vi "分层图显示1.2.1（导入色码表）.vi"(11 "IN":string) -> (3 "OUT":string)   [LabVIEW 2016]
uses:
  <vilib>/Utility/file.llb/Read Delimited Spreadsheet (DBL).vi
  <vilib>/Utility/file.llb/Read Delimited Spreadsheet (I64).vi
panel:
  in  "更换色码":bool
  in  "色码表导入":path=path "C:/Users/H301/Desktop/art闭环扫描程序/色码表/色码表（彩色2）.txt" caption="（色码表导入）"
  out "导入进度":u8(slide) scale=0.0..100.0
  in  "min":dbl format="%#_4e"
  in  "max":dbl format="%#_4e"
  in  "ESC":bool
  out "分层图":dbl[][](graph)
  in  "NEXT":bool
  in  "层数:":i32
  out "数组":dbl[][][](array[numeric])
  # "强度表"
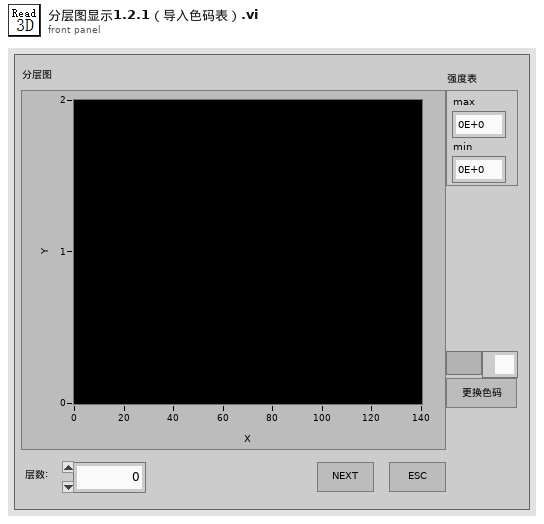
[diagram p1: front panel]
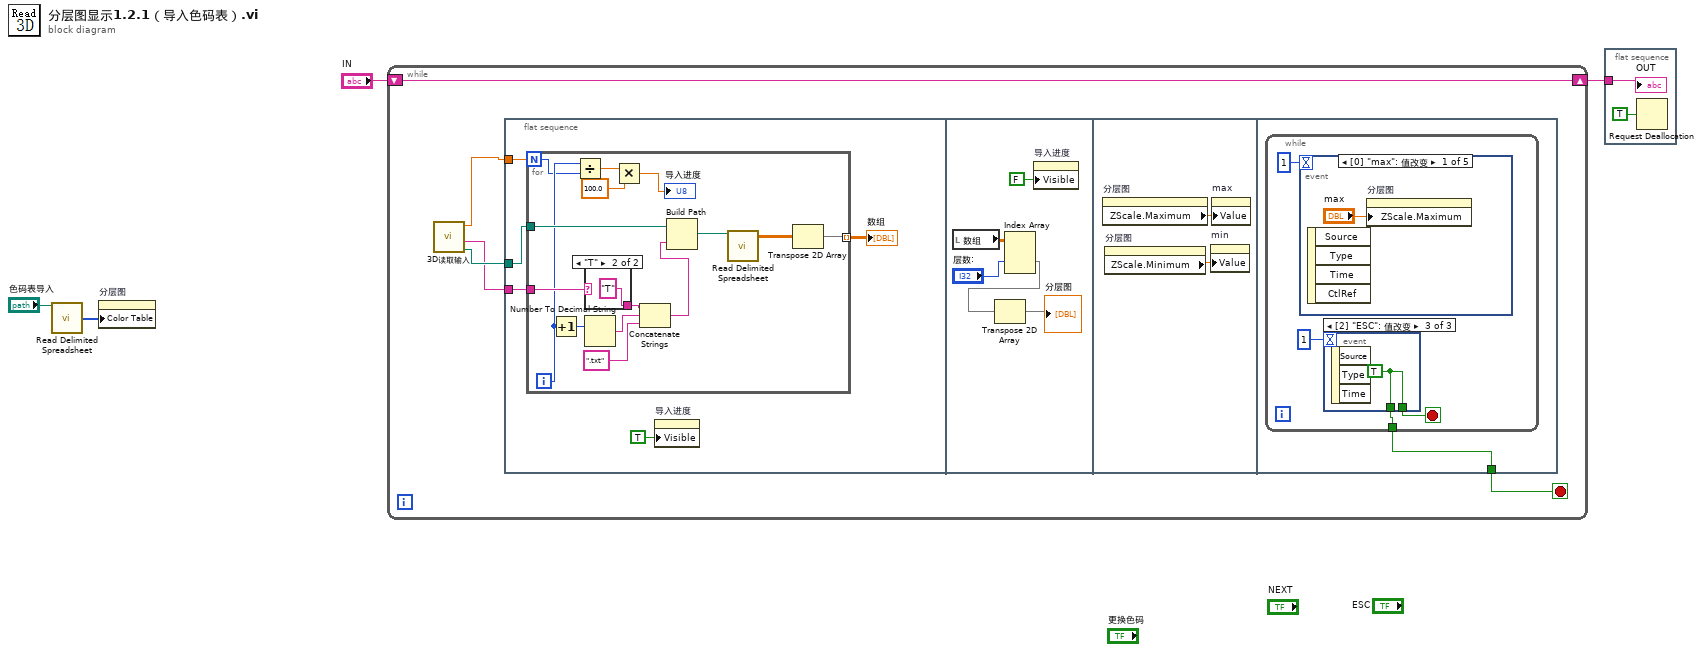
[diagram p0: block diagram]
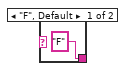
[diagram p2: hidden frame]
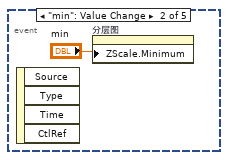
[diagram p3: hidden frame]
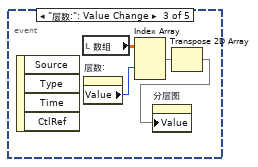
[diagram p4: hidden frame]
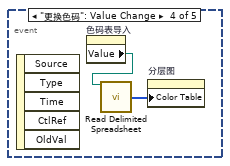
[diagram p5: hidden frame]
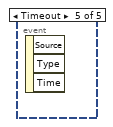
[diagram p6: hidden frame]
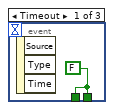
[diagram p7: hidden frame]
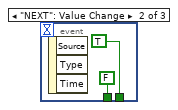
[diagram p8: hidden frame]
diagram:
  n1 = call-poly <vilib>:"Read Delimited Spreadsheet.vi"("file path (dialog if empty)"="色码表导入") -> ("first row"=w2:i64[])  [unwired: 9 in, 5 out]
  n2 = property on="分层图" class="IntGraph (严格)"("Color Table"=w2) -> ()  [unwired: 2 in, 2 out]
  n3 = while {
    shift-right: [w9] -> w3
    shift-left: "IN" -> [w9]
    stop <- w8 stop-if-true
    n4 = call "3D读取输入.vi"() -> ("文件读取路径"=w6:path, "时域谱or频域谱"=w5:string, "行总数"=w7:dbl)  [unwired: 9 in]
    n5 = flat-sequence {
      tunnel: w7 -> [w13]
      tunnel: w5 -> [w12]
      tunnel: w6 -> [w11]
      tunnel: [w39] -> w8
      frame #0 {
        n6 = for {
          N: w13 -> [w18]
          tunnel: [w28] -> w14 mode=indexing
          tunnel: w12 -> [w21]
          tunnel: w11 -> [w20]
          i -> [w19]
          n7 = Increment(x=w19) -> (x+1=w24:i32)
          n8 = Divide(x=w19, y=w18) -> (x/y=w17:dbl)
          n9 = case shown="\"T\"" w21 {
            tunnel: ["F" "T"] -> w26
            frame "F", Default {
            }
            frame "T" {
            }
          }
          n10 = Number To Decimal String(number=w24) -> (decimal integer string=w23:string)  [unwired: 1 in]
          n11 = Multiply(x=w17, y=100.0) -> (x*y=→"导入进度":dbl)
          n12 = Concatenate Strings(w26, w23, ".txt") -> (w25:string)
          n13 = Build Path(base path=w20, name or relative path=w25) -> (appended path=w27:path)
          n14 = call-poly <vilib>:"Read Delimited Spreadsheet.vi"("file path (dialog if empty)"=w27) -> ("all rows"=w29:dbl[][])  [unwired: 9 in, 5 out]
          n15 = Transpose 2D Array(2D array=w29) -> (transposed array=w28:dbl[][])
        }
        "数组" <- w14
        n16 = property on="导入进度" class="Slide (严格)"("Visible"=TRUE ("可见")) -> ()  [unwired: 2 in, 2 out]
      }
      frame #1 {
        n17 = local read "数组"() -> (w35:dbl[][][])
        n18 = Index Array(array=w35, index (dim 1)="层数:") -> (element=w33:dbl[][])  [unwired: 2 in]
        n19 = Transpose 2D Array(2D array=w33) -> (transposed array=→"分层图":dbl[][])
        n20 = property on="导入进度" class="Slide (严格)"("Visible"=FALSE ("可见")) -> ()  [unwired: 2 in, 2 out]
      }
      frame #2 {
        n21 = property on="分层图" class="IntGraph (严格)"() -> ("ZScale.Maximum"=w37:dbl)  [unwired: 2 in, 2 out]
        n22 = property on="分层图" class="IntGraph (严格)"() -> ("ZScale.Minimum"=w38:dbl)  [unwired: 2 in, 2 out]
        n23 = property on="min" class="DigNum (严格)"("Value"=w38) -> ()  [unwired: 2 in, 2 out]
        n24 = property on="max" class="DigNum (严格)"("Value"=w37) -> ()  [unwired: 2 in, 2 out]
      }
      frame #3 {
        n25 = while {
          tunnel: [w42] -> w39
          stop <- w43 stop-if-true
          n26 = event shown="[0] \"max\": 值改变" {
            selector: _ -> [_ _ _ _ _]
            dyn-events: _ -> [_ _ _ _ _]
            timeout: 1 -> [_ _ _ _ _]
            event "max": Value Change {
              n27 = event-data() -> ()  [unwired: 1 in, 4 out]
              n28 = property on="分层图" class="IntGraph (严格)"("ZScale.Maximum"="max") -> ()  [unwired: 2 in, 2 out]
            }
            event "min": Value Change {
              n29 = event-data() -> ()  [unwired: 1 in, 4 out]
              n30 = property on="分层图" class="IntGraph (严格)"("ZScale.Minimum"="min") -> ()  [unwired: 2 in, 2 out]
            }
            event "层数:": Value Change {
              n31 = event-data() -> ()  [unwired: 1 in, 4 out]
              n32 = local read "数组"() -> (w48:dbl[][][])
              n33 = property on="层数:" class="DigNum (严格)"() -> ("Value"=w49:i32)  [unwired: 2 in, 2 out]
              n34 = Index Array(array=w48, index (dim 1)=w49) -> (element=w47:dbl[][])  [unwired: 2 in]
              n35 = Transpose 2D Array(2D array=w47) -> (transposed array=w46:dbl[][])
              n36 = property on="分层图" class="IntGraph (严格)"("Value"=w46) -> ()  [unwired: 2 in, 2 out]
            }
            event "更换色码": Value Change {
              n37 = event-data() -> ()  [unwired: 1 in, 5 out]
              n38 = property on="色码表导入" class="Path"() -> ("Value"=w50:path)  [unwired: 2 in, 2 out]
              n39 = call-poly <vilib>:"Read Delimited Spreadsheet.vi"("file path (dialog if empty)"=w50) -> ("first row"=w51:i64[])  [unwired: 9 in, 5 out]
              n40 = property on="分层图" class="IntGraph (严格)"("Color Table"=w51) -> ()  [unwired: 2 in, 2 out]
            }
            event Timeout {
              n41 = event-data() -> ()  [unwired: 1 in, 3 out]
            }
          }
          n42 = event shown="[2] \"ESC\": 值改变" {
            selector: _ -> [_ _ _]
            dyn-events: _ -> [_ _ _]
            timeout: 1 -> [_ _ _]
            tunnel: [w52 TRUE w55] -> w43
            tunnel: [w52 FALSE w55] -> w42
            event Timeout {
              w52 = FALSE
              n43 = event-data() -> ()  [unwired: 1 in, 3 out]
            }
            event "NEXT": Value Change {
              n44 = event-data() -> ()  [unwired: 1 in, 3 out]
            }
            event "ESC": Value Change {
              w55 = TRUE
              n45 = event-data() -> ()  [unwired: 1 in, 3 out]
            }
          }
        }
      }
    }
  }
  n46 = flat-sequence {
    tunnel: w3 -> [w57]
    frame #0 {
      n47 = Request Deallocation(TRUE ("标志")) -> ()
      "OUT" <- w57
    }
  }
